vi "(SubVI) Get Paremeters From File Name for Passive Force Clamp Data_YCC.vi"(7 "path":path) -> (0 "Target QPD (V)":dbl, 1 "Jump (nm)":dbl, 2 "Data rate (Hz)":dbl, 3 "Moved position (um)":dbl, 4 "Laser Power (mV)":dbl, 5 "Center position (um)":dbl)   [LabVIEW 2014]
panel:
  out "after substring 2":string
  out "after substring":string
  out "before substring 3":string
  out "substring":string
  out "before substring 2":string
  out "Laser Power":string
  out "before substring":string
  in  "Tab Control":enum32{"String", "Page 2"}(tab)
  out "Center position":string
  out "Moved position":string
  out "Data rate":string
  out "Target QPD":string
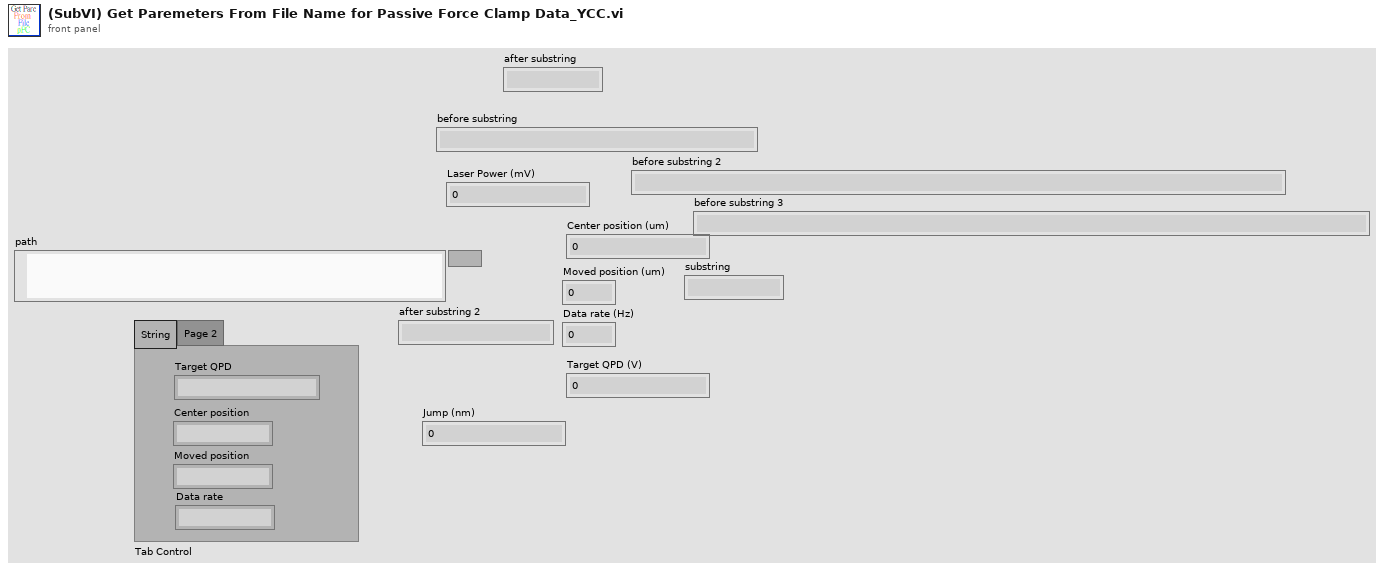
[diagram p1: front panel]
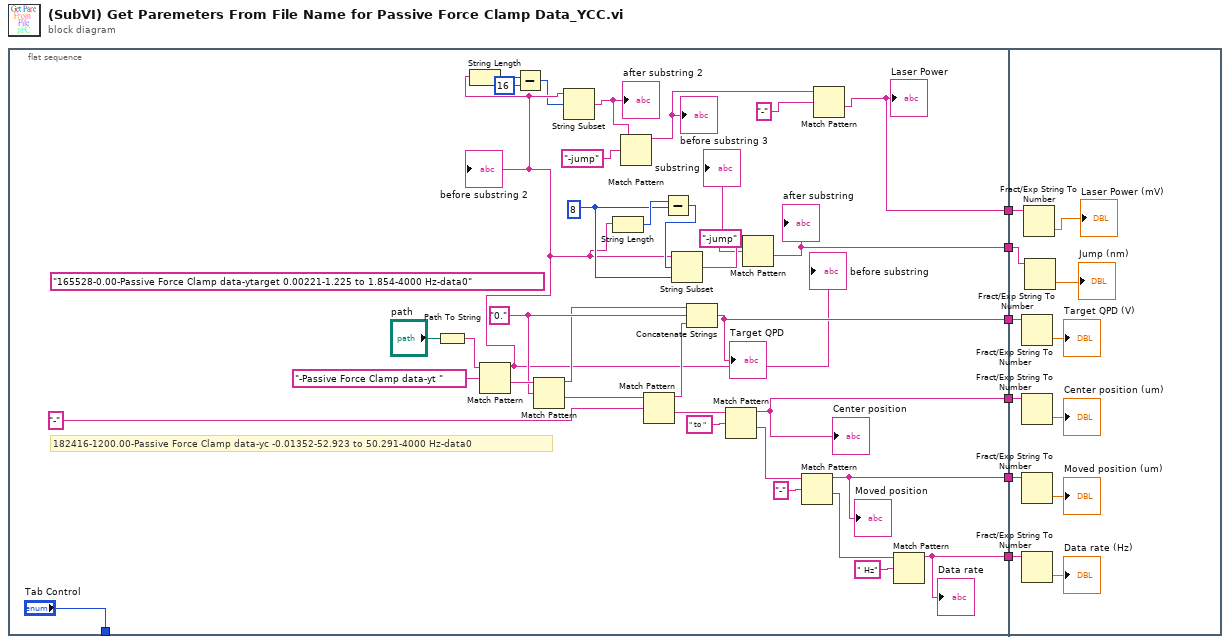
[diagram p0: block diagram]
diagram:
  n1 = flat-sequence {
    tunnel: [w35] -> w6
    tunnel: [w34] -> w5
    tunnel: [w33] -> w4
    tunnel: ["Tab Control"] -> _
    tunnel: [w24] -> w3
    tunnel: [w13] -> w2
    tunnel: [w12] -> w1
    tunnel: w6 -> [w53]
    tunnel: w5 -> [w51]
    tunnel: w4 -> [w49]
    tunnel: w3 -> [w47]
    tunnel: w2 -> [w45]
    tunnel: w1 -> [w43]
    frame #0 {
      w19 = 8 ("y")
      w26 = "0."
      (unwired) "165528-0.00-Passive Force Clamp data-ytarget 0.00221-1.225 to 1.854-4000 Hz-data0"
      # "182416-1200.00-Passive Force Clamp data-yc -0.01352-52.923 to 50.291-4000 Hz-data0"
      n2 = Path To String(path="path") -> (string=w29:string)
      n3 = Match Pattern(string=w29, regular expression="-Passive Force Clamp data-yt " ("match substring")) -> (before substring=w10:string, after substring=w31:string)  [unwired: 1 in, 2 out]
      "before substring" <- w10
      "before substring 2" <- w10
      n4 = String Length(string=w10) -> (length=w11:i32)
      n5 = Subtract(x=w11, y=16) -> (x-y=w8:i32)
      n6 = Match Pattern(string=w31, regular expression=w26) -> (before substring=w22:string, after substring=w28:string)  [unwired: 1 in, 2 out]
      n7 = String Subset(string=w10, offset (0)=w8) -> (substring=w7:string)  [unwired: 1 in]
      "after substring 2" <- w7
      n8 = String Length(string=w10) -> (length=w21:i32)
      n9 = Match Pattern(string=w7, regular expression="-jump") -> (before substring=w15:string)  [unwired: 1 in, 3 out]
      "before substring 3" <- w15
      n10 = Match Pattern(string=w28, regular expression="-") -> (before substring=w25:string, after substring=w23:string)  [unwired: 1 in, 2 out]
      n11 = Subtract(x=w21, y=w19) -> (x-y=w20:i32)
      n12 = String Subset(string=w10, offset (0)=w20, length (rest)=w19) -> (substring=w18:string)
      "substring" <- w18
      n13 = Concatenate Strings(w22, w26, w25) -> (w24:string)
      "Target QPD" <- w24
      n14 = Match Pattern(string=w23, regular expression=" to ") -> (before substring=w35:string, after substring=w39:string)  [unwired: 1 in, 2 out]
      "Center position" <- w35
      n15 = Match Pattern(string=w18, regular expression="-jump") -> (after substring=w12:string)  [unwired: 1 in, 3 out]
      "after substring" <- w12
      n16 = Match Pattern(string=w39, regular expression="-") -> (before substring=w34:string, after substring=w37:string)  [unwired: 1 in, 2 out]
      "Moved position" <- w34
      n17 = Match Pattern(string=w15, regular expression="-") -> (after substring=w13:string)  [unwired: 1 in, 3 out]
      "Laser Power" <- w13
      n18 = Match Pattern(string=w37, regular expression=" Hz") -> (before substring=w33:string)  [unwired: 1 in, 3 out]
      "Data rate" <- w33
    }
    frame #1 {
      n19 = Fract/Exp String To Number(string=w47) -> (number=→"Target QPD (V)":dbl)  [unwired: 3 in, 1 out]
      n20 = Fract/Exp String To Number(string=w53) -> (number=→"Center position (um)":dbl)  [unwired: 3 in, 1 out]
      n21 = Fract/Exp String To Number(string=w51) -> (number=→"Moved position (um)":dbl)  [unwired: 3 in, 1 out]
      n22 = Fract/Exp String To Number(string=w49) -> (number=→"Data rate (Hz)":dbl)  [unwired: 3 in, 1 out]
      n23 = Fract/Exp String To Number(string=w45) -> (number=→"Laser Power (mV)":dbl)  [unwired: 3 in, 1 out]
      n24 = Fract/Exp String To Number(string=w43) -> (number=→"Jump (nm)":dbl)  [unwired: 3 in, 1 out]
    }
  }
